vi "rvc Difference to Homogeneous Transformation.vi"(11 "Difference":dbl[](array[numeric])) -> (3 "Matrix Transformation":T1)   [LabVIEW 2013]
uses:
  <vilib>/Analysis/Matrix/Datatypes/RealMatrix.ctl
  <vilib>/Analysis/7linalg.llb/Create Special Real Matrix.vi
  <vilib>/Analysis/Matrix/Numeric/Add/Add - RM,RM.vi
  <vilib>/Analysis/NI_AALPro.lvlib
  <vilib>/Analysis/Matrix/NI_Matrix.lvlib
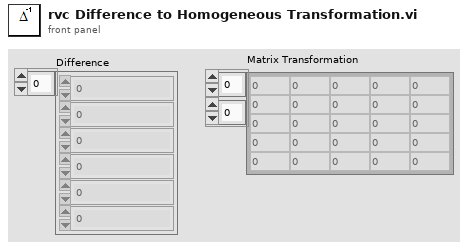
[diagram p1: front panel]
types:
  T1 = typedef "NI_Matrix.lvlib/RealMatrix.ctl" = dbl[][]
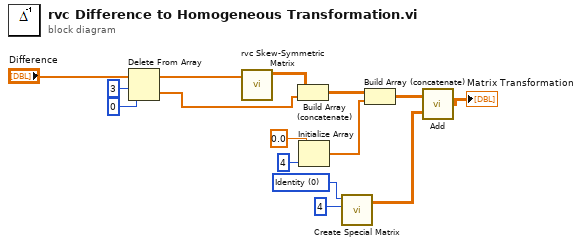
[diagram p0: block diagram]
diagram:
  w14 = 0 items=["Identity", "Diagonal", "Toeplitz", "Vandermonde", "Companion", "Hankel", "Hadamard", "Wilkinson", "Hilbert", "Inverse Hilbert", "Rosser", "Pascal"] ("matrix type")
  n1 = Delete From Array(array="Difference", length=3, index=0) -> (deleted portion=w9:dbl[], array with subset deleted=w10:dbl[])
  n2 = call "rvc Skew-Symmetric Matrix.vi"("vector"=w10) -> ("output variable"=w4:dbl[][])  [unwired: 10 in]
  n3 = Build Array (concatenate)(w4, w9) -> (w5:T1)
  n4 = Initialize Array(0.0 ("element"), 4 ("dimension size")) -> (w6:dbl[])
  n5 = call-poly <vilib>:"Create Special Matrix.vi"("matrix type"=w14, "matrix size"=4) -> ("Special Matrix"=w2:T1)  [unwired: 3 in, 1 out]
  n6 = Build Array (concatenate)(w5, w6) -> (w3:T1)
  n7 = call-poly <vilib>:"Add.vi"("Real Matrix B"=w2, "Real Matrix A"=w3) -> ("A + B"=→"Matrix Transformation":T1)
